vi "Noise Study (RT).vi"() -> ()   [LabVIEW 2013]
uses:
  <vilib>/FPGAPlugInAG/sbRIO-9626/niLvFpga_Open_sbRIO-9626.vi
  <vilib>/rvi/interface/common/dynamic/niFpgaDynamicAddResources.vi
  <vilib>/FPGAPlugInAG/Dynamic/niLvFpga_Reset_Dynamic.vi
  <vilib>/rvi/interface/common/niFpgaWaitOnOcc.vi
  <vilib>/Utility/error.llb/Error Cluster From Error Code.vi
  <vilib>/rvi/errors/niLvFpgaAdjustHostInterfaceError.vi
  <vilib>/FPGAPlugInAG/Dynamic/niLvFpga_Run_Dynamic.vi
  <vilib>/rvi/interface/nirviOpenFPGA/nirviOpenFPGA.xnode
  FPGA/bitfiles/Noise Study.lvbitx
  <vilib>/rvi/interface/nirviMethod/nirviMethod.xnode
  <vilib>/rvi/interface/nirviReadWriteControl/nirviReadWriteControl.xnode
  <vilib>/FPGAPlugInAG/Dynamic/niLvFpga_ConfigureFifo_Dynamic.vi
  <vilib>/rvi/errors/niLvFpgaMergeErrorWithErrorCode.vi
  <vilib>/FPGAPlugInAG/Dynamic/niLvFpga_ReadFifo_Dynamic.vi
  NiFpgaLv.dll
  <vilib>/rvi/interface/Simulation/niFpgaSimulationCallBeginRW.vi
  Type Defs/CAN Mode.ctl
  <vilib>/Analysis/NI_AALBase.lvlib
panel:
  out "stdev3":dbl format="%0.2f"
  out "stdev2":dbl format="%0.2f"
  out "stdev1":dbl format="%0.2f"
  in  "Stop Transfer":bool
  in  "CAN CMD":dbl
  out "element":string
  in  "stop":bool
  out "Waveform Graph":dbl[][](graph)
  in  "Pressure":dbl
  in  "index":i32 min=0 max=25 step=1
  in  "Average":bool
  in  "Filter":bool
  out "CFR":u64 format="%.0x"
  out "CFR2":u64 format="%.0x"
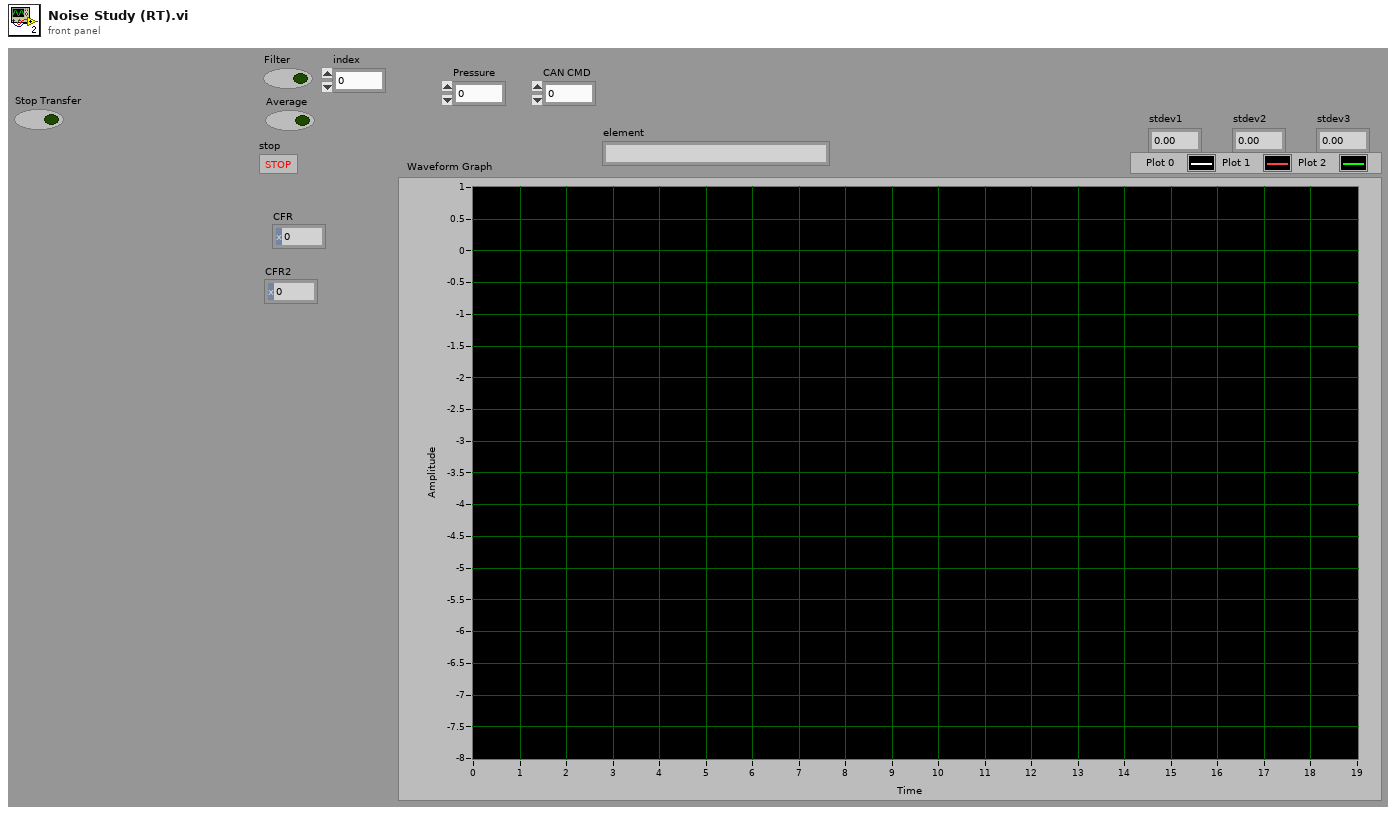
[diagram p1: front panel]
types:
  T1 = cluster{"Divide Value":u8, "Transfer Length (bits)":u8, "CS Asserted Polarity":bool, "Clock Polarity (CPOL)":bool, "Clock Phase (CPHA)":bool, "Lengthen MISO Setup":bool, "Direction Change Bit":u8, "MOSI Starts as Output":bool, "Tristatable MOSI":bool}
  T2 = typedef "CAN Mode.ctl" = enum16{"Init", "Read", "Write", "Close"}
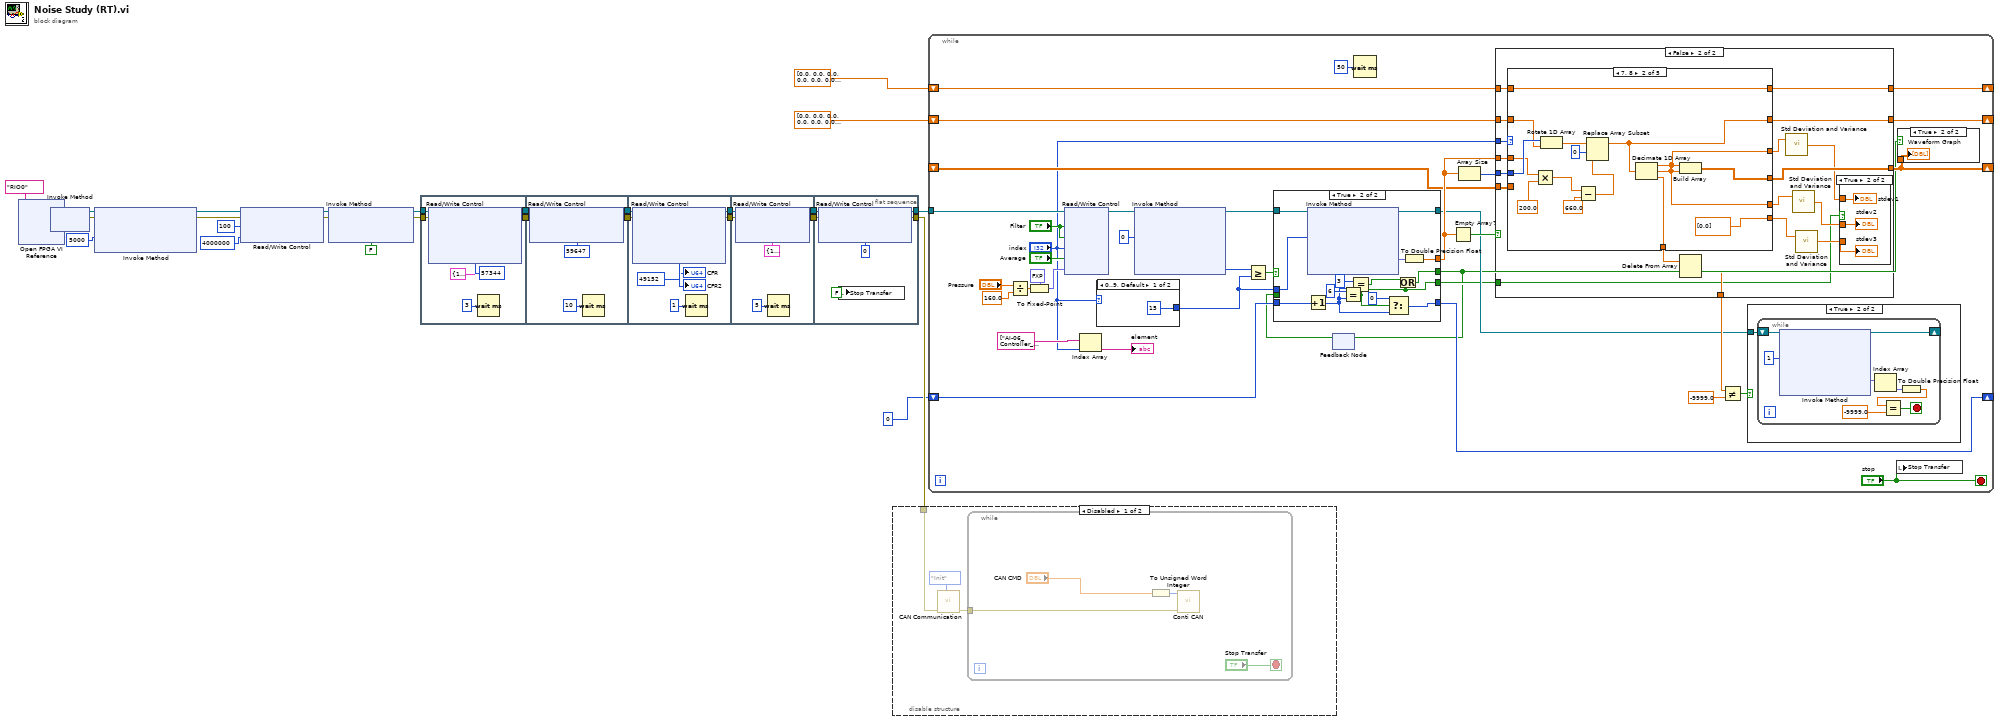
[diagram p0: block diagram]
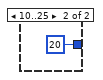
[diagram p5: hidden frame]
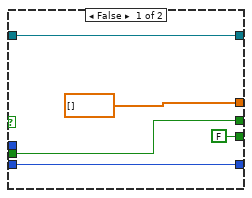
[diagram p6: hidden frame]
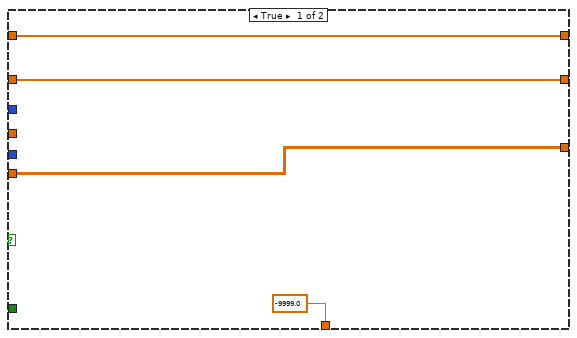
[diagram p7: hidden frame]
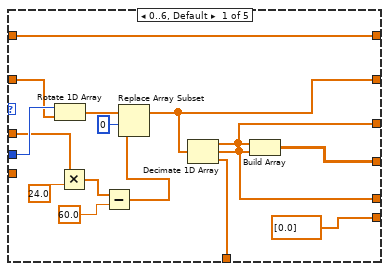
[diagram p9: hidden frame]
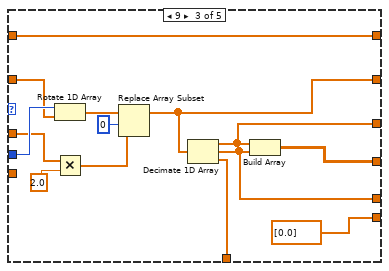
[diagram p10: hidden frame]
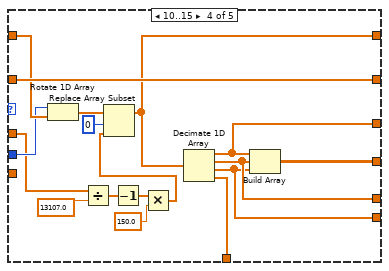
[diagram p11: hidden frame]
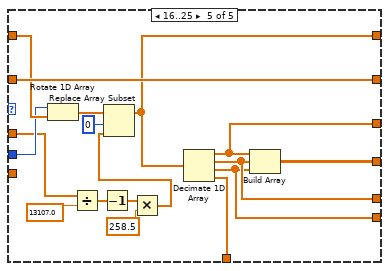
[diagram p12: hidden frame]
diagram:
  n1 = xnode "Open FPGA VI Reference"("resource name"=tag "RIO0") -> ("FPGA VI Reference Out"=w10:refnum<k20>)  [unwired: 1 in, 1 out]
  n2 = xnode "Invoke Method"("FPGA VI Reference In"=w10) -> ("FPGA VI Reference Out"=w9:refnum<k20>, "error out"=w7:errorcluster)  [unwired: 1 in]
  n3 = xnode "Invoke Method"("FPGA VI Reference In"=w9, "error in"=w7, "Requested Depth"=u32 5000) -> ("FPGA VI Reference Out"=w8:refnum<k20>, "error out"=w6:errorcluster)  [unwired: 1 out]
  n4 = xnode "Read/Write Control"("FPGA VI Reference In"=w8, "error in"=w6, "Loop Timer (uSec)"=u32 100, "AI Divisor"=u32 4000000 ("x")) -> ("FPGA VI Reference Out"=w11:refnum<k20>, "error out"=w5:errorcluster)
  n5 = xnode "Invoke Method"("FPGA VI Reference In"=w11, "error in"=w5, "Wait Until Done (F)"=FALSE) -> ("FPGA VI Reference Out"=w14:refnum<k20>, "error out"=w13:errorcluster)
  n6 = flat-sequence {
    tunnel: w14 -> [w33]
    tunnel: w13 -> [w31]
    tunnel: [w34] -> w23
    tunnel: [w32] -> w22
    tunnel: w23 -> [w39]
    tunnel: w22 -> [w38]
    tunnel: [w37] -> w21
    tunnel: [w36] -> w20
    tunnel: w21 -> [w45]
    tunnel: w20 -> [w44]
    tunnel: [w43] -> w19
    tunnel: [w42] -> w18
    tunnel: w19 -> [w53]
    tunnel: w18 -> [w52]
    tunnel: [w50] -> w17
    tunnel: [w49] -> w16
    tunnel: w17 -> [w59]
    tunnel: w16 -> [w58]
    tunnel: [w57] -> w4
    tunnel: [w55] -> w2
    frame #0 {
      w29 = T1 {"Divide Value"=1, "Transfer Length (bits)"=16, "CS Asserted Polarity"=FALSE, "Clock Polarity (CPOL)"=TRUE, "Clock Phase (CPHA)"=FALSE, "Lengthen MISO Setup"=FALSE, "Direction Change Bit"=0, "MOSI Starts as Output"=FALSE, "Tristatable MOSI"=FALSE} ("Master Settings")
      w30 = u64 57344 ("data to write")
      n7 = xnode "Read/Write Control"("FPGA VI Reference In"=w33, "error in"=w31, "AI16-23 Settings"=w29, "AI16-23 Data to Write"=w30, "AI24-31 Settings"=w29, "AI24-31 Data to Write"=w30) -> ("FPGA VI Reference Out"=w34:refnum<k20>, "error out"=w32:errorcluster)
      n8 = Wait (ms)(milliseconds to wait=u32 3) -> ()  [unwired: 1 out]
    }
    frame #1 {
      w40 = u64 59647 ("data to write")
      n9 = xnode "Read/Write Control"("FPGA VI Reference In"=w39, "error in"=w38, "AI16-23 Data to Write"=w40, "AI24-31 Data to Write"=w40) -> ("FPGA VI Reference Out"=w37:refnum<k20>, "error out"=w36:errorcluster)
      n10 = Wait (ms)(milliseconds to wait=u32 10) -> ()  [unwired: 1 out]
    }
    frame #2 {
      n11 = xnode "Read/Write Control"("FPGA VI Reference In"=w45, "error in"=w44, "AI24-31 Data to Write"=u64 49152 ("data to write")) -> ("FPGA VI Reference Out"=w43:refnum<k20>, "error out"=w42:errorcluster, "Read Data"=→"CFR":u64, "Read Data 2"=→"CFR2":u64)  [unwired: 1 in]
      n12 = Wait (ms)(milliseconds to wait=u32 1) -> ()  [unwired: 1 out]
    }
    frame #3 {
      w54 = T1 {"Divide Value"=1, "Transfer Length (bits)"=19, "CS Asserted Polarity"=FALSE, "Clock Polarity (CPOL)"=TRUE, "Clock Phase (CPHA)"=FALSE, "Lengthen MISO Setup"=FALSE, "Direction Change Bit"=0, "MOSI Starts as Output"=FALSE, "Tristatable MOSI"=FALSE} ("Master Settings")
      n13 = xnode "Read/Write Control"("FPGA VI Reference In"=w53, "error in"=w52, "AI16-23 Settings"=w54, "AI24-31 Settings"=w54) -> ("FPGA VI Reference Out"=w50:refnum<k20>, "error out"=w49:errorcluster)
      n14 = Wait (ms)(milliseconds to wait=u32 5) -> ()  [unwired: 1 out]
    }
    frame #4 {
      w60 = u64 0 ("AI16-23 Data to Write")
      n15 = xnode "Read/Write Control"("FPGA VI Reference In"=w59, "error in"=w58, "AI16-23 Data to Write"=w60, "AI24-31 Data to Write"=w60) -> ("FPGA VI Reference Out"=w57:refnum<k20>, "error out"=w55:errorcluster)
      n16 = local write "Stop Transfer"(FALSE ("Boolean")) -> ()
    }
  }
  n17 = disable-structure shown="Disabled" {
    disable-tunnel: w2 -> [w61 _]
    frame Disabled {
      n18 = call "CAN Communication.vi"("CAN Mode"=CAN_Mode."Init", "Error IN"=w61) -> ("Error OUT"=w62:errorcluster)  [unwired: 9 in]
      n19 = while {
        tunnel: w62 -> [w66]
        stop <- "Stop Transfer" stop-if-true
        n20 = To Unsigned Word Integer(number="CAN CMD") -> (unsigned 16bit integer=w65:u16)
        n21 = call "Conti CAN.vi"("Error IN"=w66, "CMD"=w65) -> ()  [unwired: 9 in, 1 out]
      }
    }
    frame Enabled {
    }
  }
  n22 = while {
    tunnel: w4 -> [w102]
    shift-right: [w91] -> _
    shift-left: dbl[] [0.0, 0.0, 0.0, 0.0, 0.0, 0.0, 0.0, 0.0, 0.0, 0.0, 0.0, 0.0, 0.0, 0.0, 0.0, 0.0, 0.0, 0.0, 0.0, 0.0, 0.0, 0.0, 0.0, 0.0, 0.0, 0.0, 0.0, 0.0, 0.0, 0.0, 0.0, 0.0, 0.0, 0.0, 0.0, 0.0, 0.0, 0.0, 0.0, 0.0, 0.0, 0.0, 0.0, 0.0, 0.0, 0.0, 0.0, 0.0, 0.0, 0.0, 0.0, 0.0, 0.0, 0.0, 0.0, 0.0, 0.0, 0.0, 0.0, 0.0, 0.0, 0.0, 0.0, 0.0, 0.0, 0.0, 0.0, 0.0, 0.0, 0.0, 0.0, 0.0, 0.0, 0.0, 0.0, 0.0, 0.0, 0.0, 0.0, 0.0] -> [w93]
    shift-right: [w90] -> _
    shift-left: dbl[] [0.0, 0.0, 0.0, 0.0, 0.0, 0.0, 0.0, 0.0, 0.0, 0.0, 0.0, 0.0, 0.0, 0.0, 0.0, 0.0, 0.0, 0.0, 0.0, 0.0, 0.0, 0.0, 0.0, 0.0, 0.0, 0.0, 0.0, 0.0, 0.0, 0.0, 0.0, 0.0, 0.0, 0.0, 0.0, 0.0, 0.0, 0.0, 0.0, 0.0, 0.0, 0.0, 0.0, 0.0, 0.0, 0.0, 0.0, 0.0, 0.0, 0.0, 0.0, 0.0, 0.0, 0.0, 0.0, 0.0, 0.0, 0.0, 0.0, 0.0] -> [w92]
    shift-right: [w85] -> _
    shift-left: _ -> [w86]
    shift-right: [w71] -> _
    shift-left: 0 -> [w72]
    stop <- "stop" stop-if-true
    n23 = Divide(x="Pressure", y=160.0) -> (x/y=w97:dbl)
    n24 = To Fixed-Point(fixed-point type=fxp<+/-,20,5> 0.0 ("AO0"), number=w97) -> (fixed-point=w94:fxp<+/-,20,5>)
    n25 = xnode "Read/Write Control"("FPGA VI Reference In"=w102, "Filter"="Filter", "Filter 2"="Filter", "index"="index", "Average"="Average", "AO0"=w94) -> ("FPGA VI Reference Out"=w101:refnum<k20>)  [unwired: 1 in, 1 out]
    n26 = Index Array(array=string[] ["AI-06_Controller_Current_1", "AI-07_Controller_Current_2", "AI-08_Controller_Current_3", "AI-09_Controller_Current_4", "AI-10_Controller_Current_5", "AI-11_Controller_Current_6", "AI-12_Spare", "AI-13_Temp_1", "AI-14_Temp_2", "AI-15_PS_Sense", "AI-16_Pump_Pressure_1", "AI-17_Pump_Pressure_2", "AI-18_Pump_Pressure_3", "AI-19_Pump_Pressure_4", "AI-20_Pump_Pressure_5", "AI-21_Pump_Pressure_6", "AI-22_Pump_Flow_1", "AI-23_Pump_Flow_2", "AI-24_Pump_Flow_3", "AI-25_Pump_Flow_4", "AI-26_Pump_Flow_5", "AI-27_Pump_Flow_6"] ("Channel Reference"), index="index") -> (element=→"element":string)
    n27 = case shown="0..9, Default" "index" {
      tunnel: [u32 15 ("y") u32 20 ("y")] -> w77
      frame 0..9, Default {
      }
      frame 10..25 {
      }
    }
    n28 = xnode "Invoke Method"("FPGA VI Reference In"=w101, "Number of Elements"=u32 0) -> ("FPGA VI Reference Out"=w103:refnum<k20>, "Elements Remaining"=w80:u32)  [unwired: 2 in, 2 out]
    n29 = Greater Or Equal?(x=w80, y=w77) -> (x >= y?=w79:bool)
    n30 = feedback #1() -> (w69:bool)  [unwired: 1 in]
    n31 = case shown="True" w79 {
      tunnel: w103 -> [w120 w135]
      tunnel: [dbl[] [] w133] -> w89
      tunnel: w77 -> [_ w132]
      tunnel: [w120 w131] -> w73
      tunnel: w72 -> [w119 w130]
      tunnel: [w119 w127] -> w71
      tunnel: [FALSE w123] -> w70
      tunnel: [w117 w122] -> w68
      tunnel: w69 -> [w117 _]
      frame False {
      }
      frame True {
        n32 = Increment(x=w130) -> (x+1=w126:i32)
        n33 = xnode "Invoke Method"("FPGA VI Reference In"=w135, "Number of Elements"=w132) -> ("FPGA VI Reference Out"=w131:refnum<k20>, "Data"=w134:fxp<+/-,28,17>[])  [unwired: 2 in, 2 out]
        n34 = Equal?(x=6, y=w126) -> (x = y?=w123:bool)
        n35 = Equal?(x=3, y=w126) -> (x = y?=w124:bool)
        n36 = Select(t=0, s=w123, f=w126) -> (s? t:f=w127:i32)
        n37 = Or(x=w124, y=w123) -> (x .or. y?=w122:bool)
        n38 = To Double Precision Float(number=w134) -> (double precision float=w133:dbl[])
      }
    }
    n39 = feedback-in #1(w68) -> ()
    n40 = Wait (ms)(milliseconds to wait=u32 50) -> ()  [unwired: 1 out]
    n41 = Empty Array?(array=w89) -> (empty?=w88:bool)
    n42 = Array Size(array=w89) -> (size(s)=w87:i32)
    n43 = case shown="False" w88 {
      tunnel: w93 -> [w139 w157]
      tunnel: w92 -> [w138 w156]
      tunnel: "index" -> [_ w155]
      tunnel: [w139 w154] -> w91
      tunnel: [w138 w153] -> w90
      tunnel: w89 -> [_ w152]
      tunnel: w87 -> [_ w151]
      tunnel: [w137 w150] -> w85
      tunnel: w86 -> [w137 w149]
      tunnel: [-9999.0 w141] -> w76
      tunnel: w70 -> [_ w140]
      frame True {
      }
      frame False {
        n44 = case shown="7, 8" w155 {
          tunnel: w157 -> [w176 w192 w206 w222 w239]
          tunnel: w156 -> [w174 w190 w204 w223 w240]
          tunnel: [w176 w192 w206 w218 w235] -> w154
          tunnel: [w171 w187 w201 w223 w240] -> w153
          tunnel: w152 -> [w169 w185 w199 w212 w229]
          tunnel: w151 -> [w175 w191 w205 w221 w238]
          tunnel: [w170 w186 w200 w217 w234] -> w150
          tunnel: w149 -> [_ _ _ _ _]
          tunnel: [w164 w180 w196 w210 w227] -> w145
          tunnel: [w163 w179 w194 w209 w226] -> w144
          tunnel: [dbl[] [0.0] dbl[] [0.0] dbl[] [0.0] w208 w225] -> w143
          tunnel: [w161 w177 w193 w207 w224] -> w142
          frame 0..6, Default {
            n45 = Rotate 1D Array(1:w174, 2:w175) -> (0:w173:dbl[])
            n46 = Multiply(x=w169, y=24.0) -> (x*y=w167:dbl[])
            n47 = Subtract(x=w167, y=60.0) -> (x-y=w165:dbl[])
            n48 = Replace Array Subset(array=w173, new element=w165, index=0) -> (w171:dbl[])
            n49 = Decimate 1D Array(w171) -> (w164:dbl[], w163:dbl[], w161:dbl[])
            n50 = Build Array(w164, w163) -> (w170:dbl[][])
          }
          frame 7, 8 {
            n51 = Multiply(x=w185, y=200.0) -> (x*y=w184:dbl[])
            n52 = Rotate 1D Array(1:w190, 2:w191) -> (0:w189:dbl[])
            n53 = Subtract(x=w184, y=660.0) -> (x-y=w183:dbl[])
            n54 = Replace Array Subset(array=w189, new element=w183, index=0) -> (w187:dbl[])
            n55 = Decimate 1D Array(w187) -> (w180:dbl[], w179:dbl[], w177:dbl[])
            n56 = Build Array(w180, w179) -> (w186:dbl[][])
          }
          frame 9 {
            n57 = Rotate 1D Array(1:w204, 2:w205) -> (0:w203:dbl[])
            n58 = Multiply(x=w199, y=2.0) -> (x*y=w198:dbl[])
            n59 = Replace Array Subset(array=w203, new element=w198, index=0) -> (w201:dbl[])
            n60 = Decimate 1D Array(w201) -> (w196:dbl[], w194:dbl[], w193:dbl[])
            n61 = Build Array(w196, w194) -> (w200:dbl[][])
          }
          frame 10..15 {
            n62 = Rotate 1D Array(1:w222, 2:w221) -> (0:w220:dbl[])
            n63 = Divide(x=w212, y=13107.0) -> (x/y=w214:dbl[])
            n64 = Decrement(x=w214) -> (x-1=w215:dbl[])
            n65 = Multiply(x=w215, y=150.0) -> (x*y=w211:dbl[])
            n66 = Replace Array Subset(array=w220, new element=w211, index=0) -> (w218:dbl[])
            n67 = Decimate 1D Array(w218) -> (w210:dbl[], w209:dbl[], w208:dbl[], w207:dbl[])
            n68 = Build Array(w210, w209, w208) -> (w217:dbl[][])
          }
          frame 16..25 {
            n69 = Rotate 1D Array(1:w239, 2:w238) -> (0:w237:dbl[])
            n70 = Divide(x=w229, y=13107.0) -> (x/y=w231:dbl[])
            n71 = Decrement(x=w231) -> (x-1=w232:dbl[])
            n72 = Multiply(x=w232, y=258.5) -> (x*y=w228:dbl[])
            n73 = Replace Array Subset(array=w237, new element=w228, index=0) -> (w235:dbl[])
            n74 = Decimate 1D Array(w235) -> (w227:dbl[], w226:dbl[], w225:dbl[], w224:dbl[])
            n75 = Build Array(w227, w226, w225) -> (w234:dbl[][])
          }
        }
        n76 = Delete From Array(array=w142) -> (deleted portion=w141:dbl)  [unwired: 2 in, 1 out]
        n77 = call <vilib>:"Std Deviation and Variance.vi"("X"=w145) -> ("standard deviation"=w148:dbl)  [unwired: 1 in, 2 out]
        n78 = call <vilib>:"Std Deviation and Variance.vi"("X"=w144) -> ("standard deviation"=w147:dbl)  [unwired: 1 in, 2 out]
        n79 = call <vilib>:"Std Deviation and Variance.vi"("X"=w143) -> ("standard deviation"=w146:dbl)  [unwired: 1 in, 2 out]
        n80 = case shown="True" w140 {
          tunnel: w148 -> [_ w160]
          tunnel: w147 -> [_ w159]
          tunnel: w146 -> [_ w158]
          frame False {
          }
          frame True {
            "stdev1" <- w160
            "stdev2" <- w159
            "stdev3" <- w158
          }
        }
      }
    }
    n81 = Not Equal?(x=w76, y=-9999.0) -> (x != y?=w74:bool)
    n82 = case shown="True" w74 {
      tunnel: w73 -> [_ w106]
      frame False {
      }
      frame True {
        n83 = while {
          shift-right: [w113] -> _
          shift-left: w106 -> [w114]
          stop <- w107 stop-if-true
          n84 = xnode "Invoke Method"("FPGA VI Reference In"=w114, "Number of Elements"=u32 1) -> ("FPGA VI Reference Out"=w113:refnum<k20>, "Data"=w111:fxp<+/-,28,17>[])  [unwired: 2 in, 2 out]
          n85 = Index Array(array=w111) -> (element=w110:fxp<+/-,28,17>)  [unwired: 1 in]
          n86 = To Double Precision Float(number=w110) -> (double precision float=w109:dbl)
          n87 = Equal?(x=w109, y=-9999.0) -> (x = y?=w107:bool)
        }
      }
    }
    n88 = local write "Stop Transfer"("stop") -> ()
    n89 = case shown="True" w68 {
      tunnel: w85 -> [_ w105]
      frame False {
      }
      frame True {
        "Waveform Graph" <- w105
      }
    }
  }
